vi "close log files.vi"(8 "error in (no error)":errorcluster, 11 "Channel in":refnum<class "SPARC4_Channel.lvclass">) -> (0 "error out":errorcluster, 3 "Channel out":refnum<class "SPARC4_Channel.lvclass">)   [LabVIEW 2018, in "SPARC4_Channel.lvclass"]
uses:
  SPARC4_Channel.lvclass
  SPARC4_Channel.lvclass/SPARC4_Channel.ctl
  Log File/Log File.lvclass
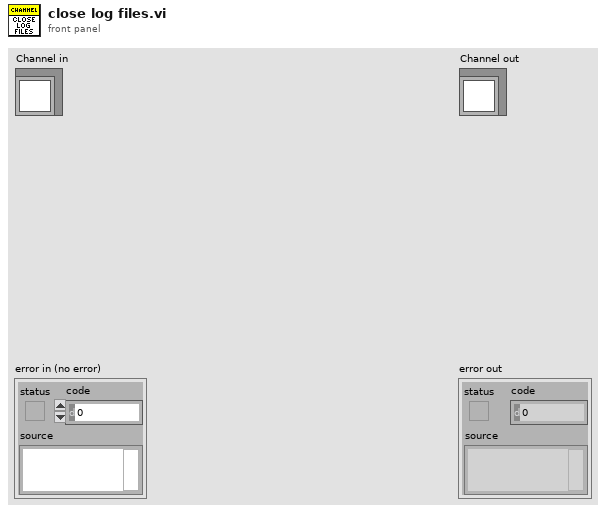
[diagram p1: front panel]
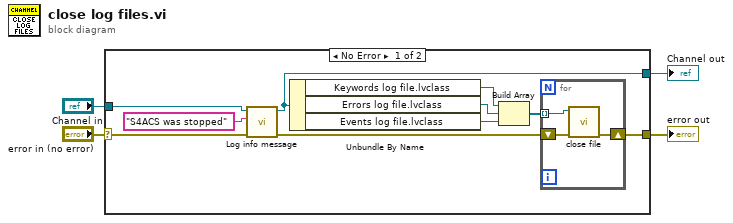
[diagram p0: block diagram]
diagram:
  n1 = case shown="No Error" "error in (no error)" {
    selector: "error in (no error)" -> [w8 w19]
    tunnel: [w11 w19] -> w3
    tunnel: [w9 w18] -> w1
    tunnel: "Channel in" -> [w10 w18]
    frame No Error {
      n2 = call "Log info message.vi"("error in (no error)"=w8, "String"="S4ACS was stopped" ("Message to log"), "Channel in"=w10) -> ("error out"=w7:errorcluster, "Channel out"=w9:refnum<class "SPARC4_Channel.lvclass">)  [unwired: 7 in]
      n3 = Unbundle By Name(w9) -> ("Keywords log file.lvclass"=w14:refnum<class "Log File.lvclass">, "Errors log file.lvclass"=w13:refnum<class "Log File.lvclass">, "Events log file.lvclass"=w5:refnum<class "Log File.lvclass">)
      n4 = Build Array(w14, w13, w5) -> (w12:refnum<class "Log File.lvclass">[])
      n5 = for {
        tunnel: w12 -> [w17] mode=indexing
        shift-right: [w15] -> w11
        shift-left: w7 -> [w16]
        n6 = call "close file.vi"("error in (no error)"=w16, "Log File in"=w17) -> ("error out"=w15:errorcluster)  [unwired: 8 in, 1 out]
      }
    }
    frame Error {
    }
  }
  "error out" <- w3
  "Channel out" <- w1
